vi "Chrg_Dschrg.vi"(0 "Data Task in":refnum<k21>, 1 "data task error in":errorcluster, 2 "#DAQ outputs (1-13)":i32, 3 "PS type":enum16{"NHR", "ITECH"}(ring), 4 "PS VISA in":refnum<visa-resource-name>, 5 "PS error in":errorcluster caption="NHR error in (no error)", 6 "DischargeCyclePath":path=path "C:/Users/ga11/Desktop/VI/results/3PtestCharge.lvm" caption="Filename", 7 "Battery Type":T1(ring), 8 "Charge/discharge":enum8{"Charge", "Discharge"}(ring), 9 "Charge/Discharge Voltage Setpoint":dbl format="%#.6g", 10 "CC or CCCV":enum16{"CC", "CCCV"}(ring), 11 "Current Setpoint":dbl format="%#.6g", 13 "Current Cutoff":dbl) -> (14 "data task out":refnum<k21>, 15 "data task error out":errorcluster, 18 "PS VIS resource name out":refnum<visa-resource-name>, 19 "PS error out":errorcluster)   [LabVIEW 2020]
uses:
  <vilib>/addons/NHR/Public/Data/Read (Ave Current).vi
  <vilib>/addons/NHR/Public/Data/Low Level/Fetch (Ave Voltage).vi
  Drivers-Essentials/NH Research Regenerative Test Series.lvlib
  Drivers-IT-M3400/IT-M3400.lvlib
panel:
  out "Read Ave Current (A)":dbl
  out "Read Ave Voltage (V)":dbl
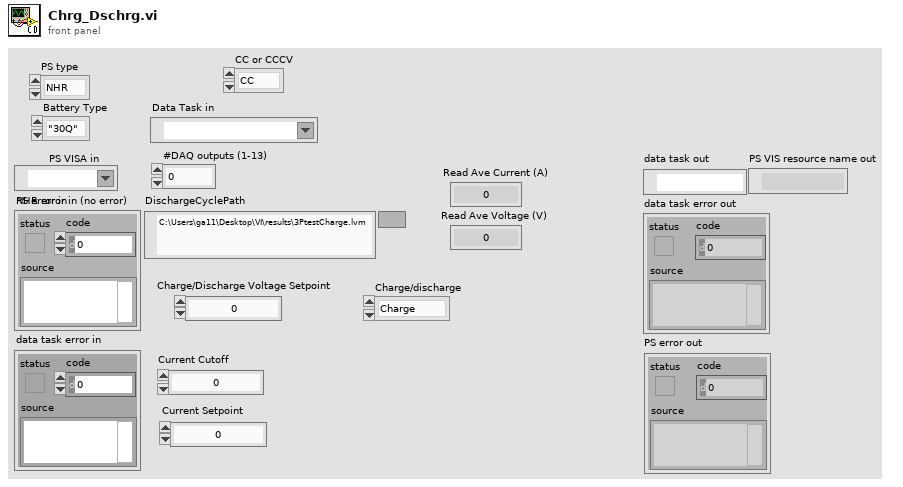
[diagram p1: front panel]
types:
  T1 = enum16{"\"30Q\"", "\"40T\"", "\"2P30Q\"", "\"3P30Q\"", "\"Nissan Leaf\""}
  T2 = cluster{"Voltage Enabled":bool, "Current Enabled":bool, "Power Enabled":bool, "Resistance Enabled":bool}
  T3 = cluster{"Baud Rate":u32, "Parity":u16, "Data Bits":u16, "Stop Bits":u16, "Flow Control":u16}
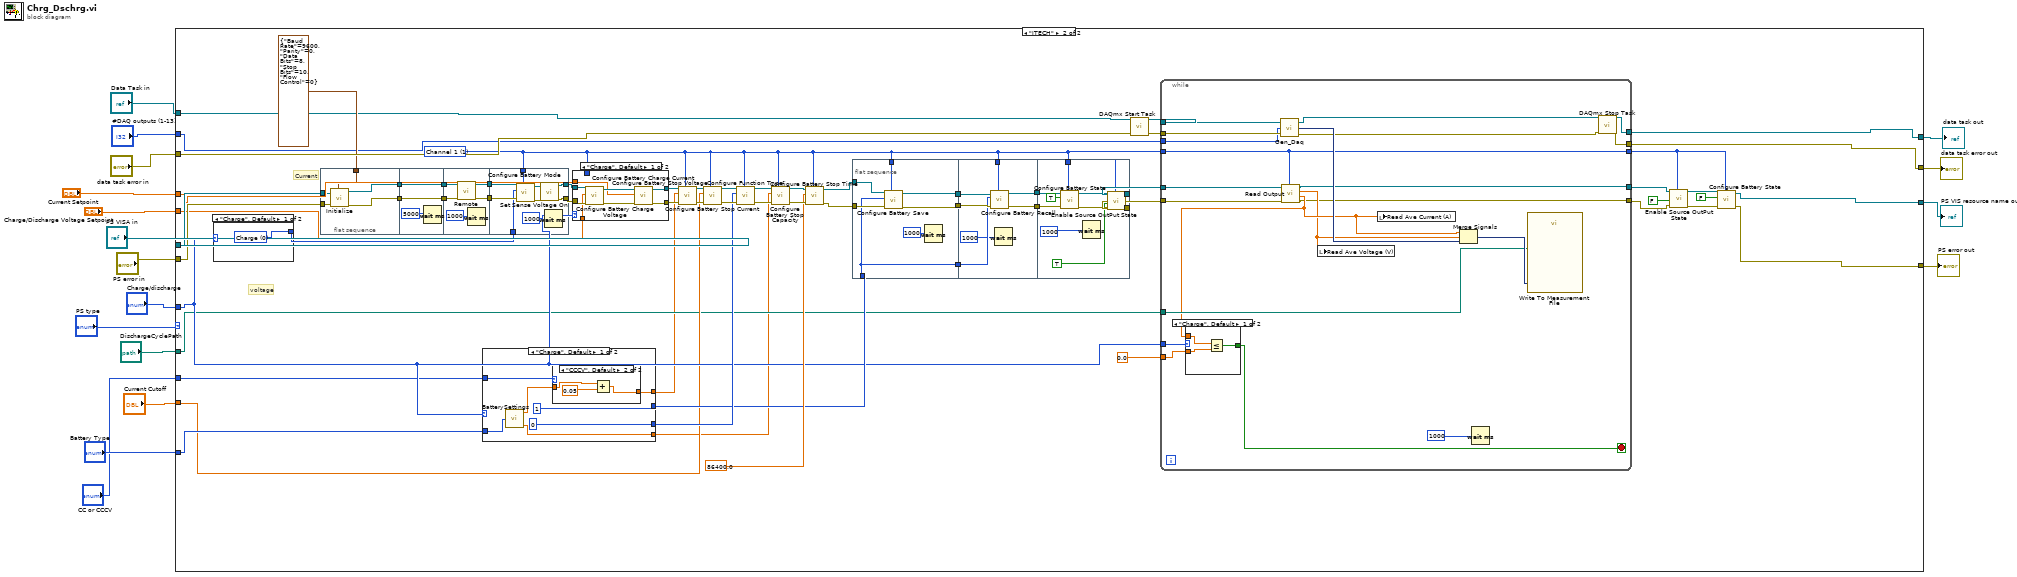
[diagram p0: block diagram]
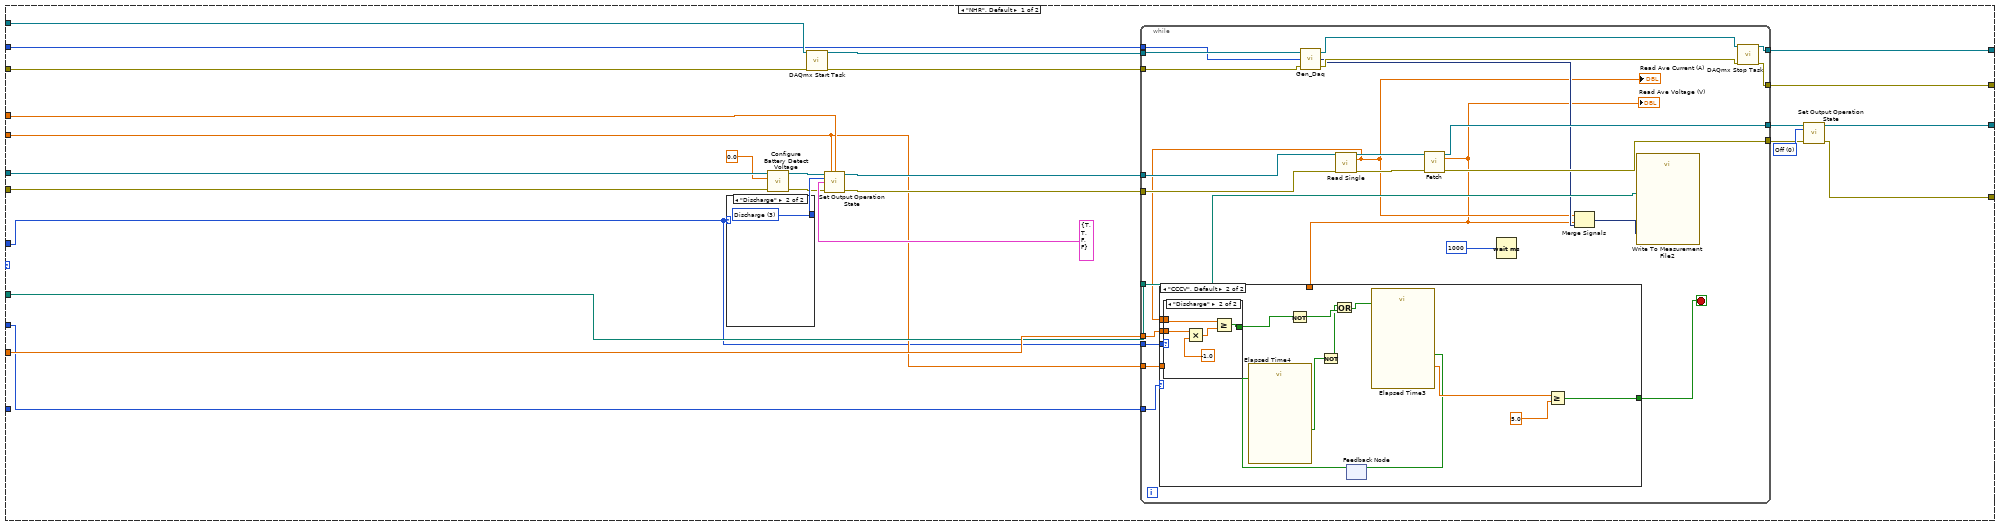
[diagram p2: hidden frame]
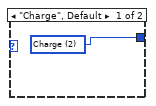
[diagram p3: hidden frame]
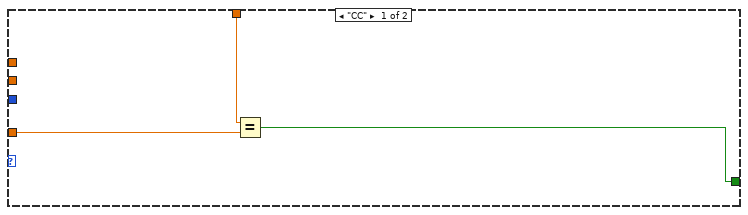
[diagram p4: hidden frame]
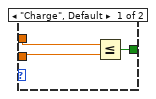
[diagram p5: hidden frame]
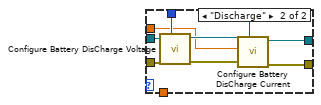
[diagram p6: hidden frame]
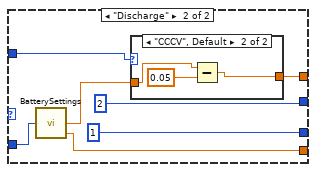
[diagram p8: hidden frame]
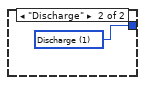
[diagram p10: hidden frame]
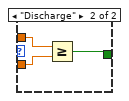
[diagram p11: hidden frame]
diagram:
  n1 = case shown="\"ITECH\"" "PS type" {
    tunnel: "Charge/Discharge Voltage Setpoint" -> [w19 w101]
    tunnel: "Current Setpoint" -> [w21 w102]
    tunnel: "Current Cutoff" -> [w42 w106]
    tunnel: "DischargeCyclePath" -> [w39 w105]
    tunnel: "Data Task in" -> [w36 w95]
    tunnel: "data task error in" -> [w35 w147]
    tunnel: "PS VISA in" -> [w31 w104]
    tunnel: "PS error in" -> [w30 w103]
    tunnel: [w28 w146] -> w9
    tunnel: [w27 w144] -> w8
    tunnel: [w26 w145] -> w7
    tunnel: [w25 w143] -> w6
    tunnel: "#DAQ outputs (1-13)" -> [w22 w110]
    tunnel: "Battery Type" -> [_ w107]
    tunnel: "Charge/discharge" -> [w18 w108]
    tunnel: "CC or CCCV" -> [w20 w100]
    frame "NHR", Default {
      w34 = 0 items=["Off", "Standby", "Charge", "Discharge", "Battery"] ("Mode (0: Off)")
      n2 = case shown="\"Discharge\"" w18 {
        tunnel: [w45 w46] -> w40
        frame "Charge", Default {
          w45 = 2 items=["Off", "Standby", "Charge", "Discharge", "Battery"] ("Mode (0: Off)")
        }
        frame "Discharge" {
          w46 = 3 items=["Off", "Standby", "Charge", "Discharge", "Battery"] ("Mode (0: Off)")
        }
      }
      n3 = call <vilib>:"Configure Battery Detect Voltage.vi"("VISA resource name"=w31, "Battery Detect Voltage (0V)"=0.0, "error in (no error)"=w30) -> ("VISA resource name out"=w33:refnum<visa-resource-name>, "error out"=w32:errorcluster)  [unwired: 11 in]
      n4 = call <vilib>:"DAQmx Start Task.vi"("task/channels in"=w36, "error in"=w35) -> ("task out"=w38:refnum<k21>, "error out"=w37:errorcluster)  [unwired: 12 in]
      n5 = call "Set Output Operation State.vi"("VISA resource name"=w33, "Voltage Setpoint (0 V)"=w19, "Current Setpoint (0 A)"=w21, "Mode (0: Off)"=w40, "Enable"=T2 {"Voltage Enabled"=TRUE, "Current Enabled"=TRUE, "Power Enabled"=FALSE, "Resistance Enabled"=FALSE}, "error in (no error)"=w32) -> ("VISA resource name out"=w44:refnum<visa-resource-name>, "error out"=w43:errorcluster)  [unwired: 8 in]
      n6 = while {
        tunnel: w44 -> [w68]
        tunnel: w43 -> [w67]
        tunnel: w42 -> [w52]
        tunnel: w37 -> [w57]
        tunnel: w38 -> [w58]
        tunnel: w39 -> [w63]
        tunnel: [w62] -> w28
        tunnel: [w61] -> w26
        tunnel: [w60] -> w24
        tunnel: [w59] -> w23
        tunnel: w22 -> [w56]
        tunnel: w20 -> [w50]
        tunnel: w19 -> [w48]
        tunnel: w18 -> [w47]
        stop <- w64 stop-if-true
        n7 = call "Gen_Daq.vi"("error in"=w57, "#DAQ outputs (1-13)"=w56, "task/channels in"=w58) -> ("error out"=w54:errorcluster, "DaQ_output"=w53:dynamicdata, "task out"=w55:refnum<k21>)
        n8 = call-poly "Read Single.vi"("VISA resource name"=w68, "error in (no error)"=w67) -> ("VISA resource name out"=w69:refnum<visa-resource-name>, "Ave Current (A)"=w51:dbl, "error out"=w70:errorcluster)  [unwired: 11 in]
        "Read Ave Current (A)" <- w51
        n9 = call-poly "Fetch.vi"("VISA resource name"=w69, "error in (no error)"=w70) -> ("VISA resource name out"=w60:refnum<visa-resource-name>, "Ave Voltage (V)"=w49:dbl, "error out"=w59:errorcluster)  [unwired: 11 in]
        "Read Ave Voltage (V)" <- w49
        n10 = case shown="\"CCCV\", Default" w50 {
          tunnel: [w71 w80] -> w64
          tunnel: w52 -> [_ w77]
          tunnel: w51 -> [_ w76]
          tunnel: w49 -> [w73 _]
          tunnel: w48 -> [w72 _]
          tunnel: w47 -> [_ w74]
          frame "CC" {
            n11 = Equal?(x=w73, y=w72) -> (x = y?=w71:bool)
          }
          frame "CCCV", Default {
            n12 = case shown="\"Discharge\"" w74 {
              tunnel: w77 -> [w88 w93]
              tunnel: w76 -> [w89 w91]
              tunnel: [w87 w90] -> w75
              frame "Charge", Default {
                n13 = Less Or Equal?(x=w89, y=w88) -> (x <= y?=w87:bool)
              }
              frame "Discharge" {
                n14 = Multiply(x=w93, y=-1.0) -> (x*y=w92:dbl)
                n15 = Greater Or Equal?(x=w91, y=w92) -> (x >= y?=w90:bool)
              }
            }
            n16 = Not(x=w75) -> (.not. x?=w86:bool)
            n17 = feedback #1() -> (w78:bool)  [unwired: 1 in]
            n18 = call "Elapsed Time4"("Reset"=w78) -> ("Time has Elapsed"=w85:bool)  [unwired: 11 in, 7 out]
            n19 = Not(x=w85) -> (.not. x?=w84:bool)
            n20 = Or(x=w84, y=w86) -> (x .or. y?=w83:bool)
            n21 = call "Elapsed Time3"("Reset"=w83) -> ("Elapsed Time (s)"=w82:dbl, "Time has Elapsed"=w79:bool)  [unwired: 11 in, 6 out]
            n22 = feedback-in #1(w79) -> ()
            n23 = Greater Or Equal?(x=w82, y=5.0) -> (x >= y?=w80:bool)
          }
        }
        n24 = Wait (ms)(milliseconds to wait=1000) -> ()  [unwired: 1 out]
        n25 = Merge Signals "Merge Signals"(w51, w49, w53) -> (w66:dynamicdata)
        n26 = call "Write To Measurement File2"("Signals"=w66, "Filename"=w63) -> ()  [unwired: 15 in, 3 out]
        n27 = call <vilib>:"DAQmx Stop Task.vi"("task/channels in"=w55, "error in"=w54) -> ("task out"=w62:refnum<k21>, "error out"=w61:errorcluster)  [unwired: 12 in]
      }
      n28 = call "Set Output Operation State.vi"("VISA resource name"=w24, "Mode (0: Off)"=w34, "error in (no error)"=w23) -> ("VISA resource name out"=w27:refnum<visa-resource-name>, "error out"=w25:errorcluster)  [unwired: 11 in]
    }
    frame "ITECH" {
      w111 = 1 items=["Channel 1"=1, "Channel 2"=2, "Channel 3"=3, "Channel 4"=4, "Channel 5"=5, "Channel 6"=6, "Channel 7"=7, "Channel 8"=8, "Channel 8"=9, "Channel 10"=10, "Channel 11"=11, "Channel 12"=12, "Channel 13"=13, "Channel 14"=14, "Channel 15"=15, "Channel 16"=16] ("Channel")
      # "voltage"
      # "Current"
      n29 = case shown="\"Charge\", Default" w108 {
        tunnel: [w240 w241] -> w121
        frame "Charge", Default {
          w240 = u8 0 items=["Charge", "Discharge"] ("Battery Mode")
        }
        frame "Discharge" {
          w241 = u8 1 items=["Charge", "Discharge"] ("Battery Mode")
        }
      }
      n30 = flat-sequence {
        tunnel: [w156] -> w136
        tunnel: [w157] -> w135
        tunnel: T3 {"Baud Rate"=9600, "Parity"=0, "Data Bits"=8, "Stop Bits"=10, "Flow Control"=0} ("Serial Configuration") -> [w160]
        tunnel: w103 -> [w159]
        tunnel: w104 -> [w158]
        tunnel: w136 -> [w163]
        tunnel: [w163] -> w134
        tunnel: w135 -> [w162]
        tunnel: [w162] -> w133
        tunnel: [w168] -> w132
        tunnel: [w167] -> w131
        tunnel: w134 -> [w166]
        tunnel: w133 -> [w165]
        tunnel: w132 -> [w174]
        tunnel: w131 -> [w176]
        tunnel: w111 -> [w177]
        tunnel: w121 -> [w175]
        tunnel: [w170] -> w97
        tunnel: [w169] -> w96
        frame #0 {
          n31 = call <instrlib>:"Initialize.vi"("Serial Configuration"=w160, "error in"=w159, "VISA resource name"=w158) -> ("error out"=w157:errorcluster, "VISA resource name out"=w156:refnum<visa-resource-name>)  [unwired: 7 in]
        }
        frame #1 {
          n32 = Wait (ms)(milliseconds to wait=5000) -> ()  [unwired: 1 out]
        }
        frame #2 {
          n33 = call <instrlib>:"Remote.vi"("error in"=w165, "VISA resource name"=w166) -> ("error out"=w167:errorcluster, "VISA resource name out"=w168:refnum<visa-resource-name>)  [unwired: 8 in]
          n34 = Wait (ms)(milliseconds to wait=1000) -> ()  [unwired: 1 out]
        }
        frame #3 {
          n35 = call "Configure Battery Mode.vi"("Channel"=w177, "error in"=w176, "Battery Mode"=w175, "VISA resource name"=w174) -> ("error out"=w171:errorcluster, "VISA resource name out"=w172:refnum<visa-resource-name>)  [unwired: 6 in]
          n36 = call "Set Sense Voltage On.vi"("error in"=w171, "VISA resource name"=w172) -> ("error out"=w170:errorcluster, "VISA resource name out"=w169:refnum<visa-resource-name>)  [unwired: 8 in]
          n37 = Wait (ms)(milliseconds to wait=1000) -> ()  [unwired: 1 out]
        }
      }
      n38 = case shown="\"Charge\", Default" w108 {
        tunnel: w107 -> [w224 w235]
        tunnel: [u8 0 ("File") u8 1 ("File")] -> w115
        tunnel: [u8 1 ("File") u8 2 ("File")] -> w114
        tunnel: [w221 w232] -> w98
        tunnel: w100 -> [w218 w231]
        tunnel: [w219 w230] -> w99
        frame "Charge", Default {
          n39 = call "BatterySettings.vi"("Battery Type"=w224) -> ("RatedCapacity (Ah)"=w221:dbl, "Max Voltage (V)"=w220:dbl)  [unwired: 2 in, 1 out]
          n40 = case shown="\"CCCV\", Default" w218 {
            tunnel: w220 -> [w225 w227]
            tunnel: [w225 w226] -> w219
            frame "CC" {
            }
            frame "CCCV", Default {
              n41 = Add(x=w227, y=0.05) -> (x+y=w226:dbl)
            }
          }
        }
        frame "Discharge" {
          n42 = call "BatterySettings.vi"("Battery Type"=w235) -> ("RatedCapacity (Ah)"=w232:dbl, "Min Voltage (V)"=w229:dbl)  [unwired: 2 in, 1 out]
          n43 = case shown="\"CCCV\", Default" w231 {
            tunnel: w229 -> [w236 w238]
            tunnel: [w236 w237] -> w230
            frame "CC" {
            }
            frame "CCCV", Default {
              n44 = Subtract(x=w238, y=0.05) -> (x-y=w237:dbl)
            }
          }
        }
      }
      n45 = case shown="\"Charge\", Default" w108 {
        tunnel: w96 -> [w202 w217]
        tunnel: w97 -> [w209 w216]
        tunnel: [w205 w213] -> w126
        tunnel: [w204 w212] -> w125
        tunnel: w111 -> [_ w211]
        tunnel: w102 -> [w206 w210]
        tunnel: w101 -> [w203 _]
        frame "Charge", Default {
          n46 = call "Configure Battery Charge Voltage.vi"("error in"=w209, "Charge Voltage(V)"=w203, "VISA resource name"=w202) -> ("error out"=w207:errorcluster, "VISA resource name out"=w208:refnum<visa-resource-name>)  [unwired: 6 in]
          n47 = call "Configure Battery Charge Current.vi"("error in"=w207, "Charge Current(A)"=w206, "VISA resource name"=w208) -> ("error out"=w204:errorcluster, "VISA resource name out"=w205:refnum<visa-resource-name>)  [unwired: 7 in]
        }
        frame "Discharge" {
          n48 = call "Configure Battery DisCharge Voltage.vi"("Channel"=w211, "error in"=w216, "VISA resource name"=w217) -> ("error out"=w214:errorcluster, "VISA resource name out"=w215:refnum<visa-resource-name>)  [unwired: 7 in]
          n49 = call "Configure Battery DisCharge Current.vi"("Channel"=w211, "error in"=w214, "Discharge Current(A)"=w210, "VISA resource name"=w215) -> ("error out"=w212:errorcluster, "VISA resource name out"=w213:refnum<visa-resource-name>)  [unwired: 6 in]
        }
      }
      n50 = call "Configure Battery Stop Voltage.vi"("Channel"=w111, "error in"=w125, "Stop Voltage(V)"=w99, "VISA resource name"=w126) -> ("error out"=w129:errorcluster, "VISA resource name out"=w130:refnum<visa-resource-name>)  [unwired: 6 in]
      n51 = call "Configure Battery Stop Current.vi"("Channel"=w111, "error in"=w129, "Stop Current(A)"=w106, "VISA resource name"=w130) -> ("error out"=w117:errorcluster, "VISA resource name out"=w119:refnum<visa-resource-name>)  [unwired: 6 in]
      n52 = call "Configure Function Type.vi"("Channel"=w111, "error in"=w117, "Function Type"=w115, "VISA resource name"=w119) -> ("error out"=w116:errorcluster, "VISA resource name out"=w118:refnum<visa-resource-name>)  [unwired: 6 in]
      n53 = call "Configure Battery Stop Capacity.vi"("Channel"=w111, "error in"=w116, "Stop Capacity(Ah)"=w98, "VISA resource name"=w118) -> ("error out"=w127:errorcluster, "VISA resource name out"=w128:refnum<visa-resource-name>)  [unwired: 6 in]
      n54 = call "Configure Battery Stop Time.vi"("Channel"=w111, "error in"=w127, "Stop Time(S)"=86400.0, "VISA resource name"=w128) -> ("error out"=w123:errorcluster, "VISA resource name out"=w122:refnum<visa-resource-name>)  [unwired: 6 in]
      n55 = flat-sequence {
        tunnel: w114 -> [w183]
        tunnel: w111 -> [w178]
        tunnel: [w181] -> w141
        tunnel: [w183] -> w140
        tunnel: [w180] -> w139
        tunnel: w123 -> [w184]
        tunnel: w122 -> [w182]
        tunnel: [w187] -> w138
        tunnel: [w188] -> w137
        tunnel: w141 -> [w191]
        tunnel: w140 -> [w190]
        tunnel: w139 -> [w189]
        tunnel: w111 -> [w185]
        tunnel: [w195] -> w113
        tunnel: [w194] -> w112
        tunnel: w111 -> [w193]
        tunnel: w138 -> [w201]
        tunnel: w137 -> [w200]
        frame #0 {
          n56 = call "Configure Battery Save.vi"("Channel"=w178, "error in"=w184, "File"=w183, "VISA resource name"=w182) -> ("error out"=w181:errorcluster, "VISA resource name out"=w180:refnum<visa-resource-name>)  [unwired: 6 in]
          n57 = Wait (ms)(milliseconds to wait=1000) -> ()  [unwired: 1 out]
        }
        frame #1 {
          n58 = call "Configure Battery Recall.vi"("Channel"=w185, "error in"=w191, "File"=w190, "VISA resource name"=w189) -> ("error out"=w188:errorcluster, "VISA resource name out"=w187:refnum<visa-resource-name>)  [unwired: 6 in]
          n59 = Wait (ms)(milliseconds to wait=1000) -> ()  [unwired: 1 out]
        }
        frame #2 {
          n60 = call "Configure Battery State.vi"("Channel"=w193, "error in"=w200, "State"=TRUE, "VISA resource name"=w201) -> ("error out"=w198:errorcluster, "VISA resource name out"=w199:refnum<visa-resource-name>)  [unwired: 6 in]
          n61 = Wait (ms)(milliseconds to wait=1000) -> ()  [unwired: 1 out]
          n62 = call "Enable Source OutPut State.vi"("Channel"=w193, "error in"=w198, "State"=TRUE ("Enable Output|Intput"), "VISA resource name"=w199) -> ("error out"=w194:errorcluster, "VISA resource name out"=w195:refnum<visa-resource-name>)  [unwired: 6 in]
        }
      }
      n63 = call <vilib>:"DAQmx Start Task.vi"("task/channels in"=w95, "error in"=w147) -> ("task out"=w149:refnum<k21>, "error out"=w148:errorcluster)  [unwired: 12 in]
      n64 = while {
        tunnel: [w243] -> w151
        tunnel: [w242] -> w150
        tunnel: w149 -> [w261]
        tunnel: w148 -> [w260]
        tunnel: [w257] -> w146
        tunnel: [w256] -> w145
        tunnel: 0.0 -> [w253]
        tunnel: w113 -> [w244]
        tunnel: w112 -> [w245]
        tunnel: w111 -> [w248]
        tunnel: w110 -> [w251]
        tunnel: [w248] -> w109
        tunnel: w108 -> [w250]
        tunnel: w105 -> [w249]
        stop <- w252 stop-if-true
        n65 = call "Gen_Daq.vi"("error in"=w260, "#DAQ outputs (1-13)"=w251, "task/channels in"=w261) -> ("error out"=w258:errorcluster, "DaQ_output"=w262:dynamicdata, "task out"=w259:refnum<k21>)
        n66 = call "Read Output.vi"("Channel"=w248, "error in"=w245, "VISA resource name"=w244) -> ("error out"=w242:errorcluster, "Read Current(A)"=w247:dbl, "Read Voltage(V)"=w246:dbl, "VISA resource name out"=w243:refnum<visa-resource-name>)  [unwired: 5 in]
        n67 = case shown="\"Charge\", Default" w250 {
          tunnel: w253 -> [w264 w267]
          tunnel: w247 -> [w265 w268]
          tunnel: [w263 w266] -> w252
          frame "Charge", Default {
            n68 = Less Or Equal?(x=w265, y=w264) -> (x <= y?=w263:bool)
          }
          frame "Discharge" {
            n69 = Greater Or Equal?(x=w268, y=w267) -> (x >= y?=w266:bool)
          }
        }
        n70 = local write "Read Ave Voltage (V)"(w246) -> ()
        n71 = local write "Read Ave Current (A)"(w247) -> ()
        n72 = Merge Signals "Merge Signals"(w247, w246, w262) -> (w255:dynamicdata)
        n73 = Wait (ms)(milliseconds to wait=1000) -> ()  [unwired: 1 out]
        n74 = call "Write To Measurement File"("Signals"=w255, "Filename"=w249) -> ()  [unwired: 15 in, 3 out]
        n75 = call <vilib>:"DAQmx Stop Task.vi"("task/channels in"=w259, "error in"=w258) -> ("task out"=w257:refnum<k21>, "error out"=w256:errorcluster)  [unwired: 12 in]
      }
      n76 = call "Enable Source OutPut State.vi"("Channel"=w109, "error in"=w150, "State"=FALSE, "VISA resource name"=w151) -> ("error out"=w154:errorcluster, "VISA resource name out"=w155:refnum<visa-resource-name>)  [unwired: 6 in]
      n77 = call "Configure Battery State.vi"("Channel"=w109, "error in"=w154, "State"=FALSE, "VISA resource name"=w155) -> ("error out"=w143:errorcluster, "VISA resource name out"=w144:refnum<visa-resource-name>)  [unwired: 6 in]
    }
  }
  "data task out" <- w9
  "PS VIS resource name out" <- w8
  "data task error out" <- w7
  "PS error out" <- w6
